vi "add_Header.vi"(3 "reset seq?":bool, 4 "frame_id":string, 5 "msg in":string) -> (2 "msg out":string)   [LabVIEW 2012]
uses:
  <userlib>/rosforlv/ROS/MessageBuilding/std_msgs/subs/u32Scalar.vi
  <userlib>/rosforlv/ROS/MessageBuilding/std_msgs/subs/timeScalar.vi
  <userlib>/rosforlv/ROS/MessageBuilding/std_msgs/subs/stringScalar.vi
panel:
  out "Ros Header":T1
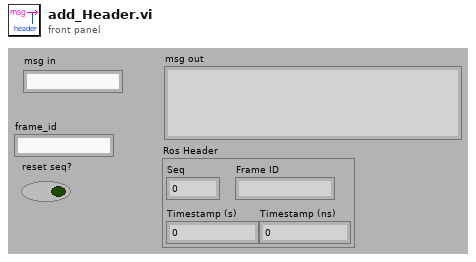
[diagram p1: front panel]
types:
  T1 = cluster{"Seq":u32, "Timestamp (s)":i32, "Frame ID":string, "Timestamp (ns)":i32}
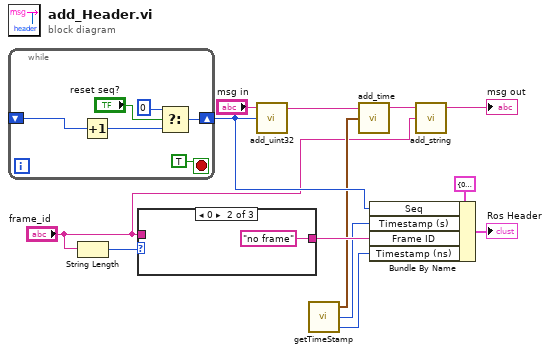
[diagram p0: block diagram]
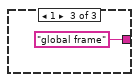
[diagram p3: hidden frame]
diagram:
  n1 = while {
    shift-right: [w15] -> w7
    shift-left: _ -> [w18]
    stop <- TRUE stop-if-true
    n2 = Increment(x=w18) -> (x+1=w14:u32)
    n3 = Select(t=u32 0, s="reset seq?", f=w14) -> (s? t:f=w15:u32)
  }
  n4 = String Length(string="frame_id") -> (length=w12:i32)
  n5 = case shown="0" w12 {
    tunnel: [w20 "no frame" ("frame_id") "global frame" ("frame_id")] -> w11
    tunnel: "frame_id" -> [w20 _ _]
    frame Default {
    }
    frame 0 {
    }
    frame 1 {
    }
  }
  n6 = call-poly <userlib>:"add_uint32.vi"("Numeric"=w7, "msg in"="msg in") -> ("msg out"=w4:string)  [unwired: 3 in]
  n7 = call <userlib>:"getTimeStamp.vi"() -> ("nsecs"=w8:i32, "secs"=w9:i32, "ROS Time"=w6:cluster{"secs":i32, "nsecs":i32})  [unwired: 2 in]
  n8 = call-poly <userlib>:"add_time.vi"("Time"=w6, "msg in"=w4) -> ("msg out"=w3:string)  [unwired: 3 in]
  n9 = Bundle By Name(cluster=T1 {"Seq"=0, "Timestamp (s)"=0, "Frame ID"="", "Timestamp (ns)"=0} ("ROS Msg Header"), "Seq"=w7, "Timestamp (s)"=w9, "Frame ID"=w11, "Timestamp (ns)"=w8) -> (→"Ros Header":T1)
  n10 = call-poly <userlib>:"add_string.vi"("String"="frame_id", "msg in"=w3) -> ("msg out"=→"msg out":string)  [unwired: 3 in]
